vi "While Loop VI.vi"() -> ()   [LabVIEW 2020]
panel:
  out "Loop Iterations":i32
  in  "stop":bool
  in  "Value":dbl
  # "While Loop"
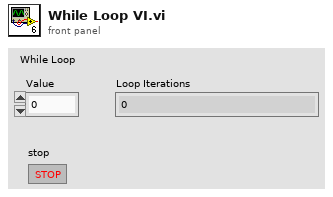
[diagram p1: front panel]
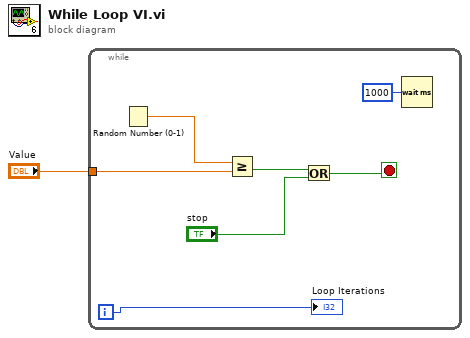
[diagram p0: block diagram]
diagram:
  n1 = while {
    tunnel: "Value" -> [w7]
    i -> [w4]
    stop <- w5 stop-if-true
    n2 = Random Number (0-1)() -> (number: 0 to 1=w8:dbl)
    n3 = Greater Or Equal?(x=w8, y=w7) -> (x >= y?=w6:bool)
    n4 = Or(x=w6, y="stop") -> (x .or. y?=w5:bool)
    n5 = Wait (ms)(milliseconds to wait=u32 1000) -> ()  [unwired: 1 out]
    "Loop Iterations" <- w4
  }
